vi "SetScrapped.vi"(8 "error in":errorcluster, 10 "Srapped":bool, 11 "ProductUnit in":refnum<class "ProductUnit.lvclass">) -> (0 "error out":errorcluster, 3 "ProductUnit out":refnum<class "ProductUnit.lvclass">)   [LabVIEW 2021, in "ProligentXMLGenerator.lvlib" / "ProductUnit.lvclass"]
doc: "Flag representing whether the product unit has been scrapped or not. When not specified, it is assumed that the product unit is not scrapped."
uses:
  ProductUnit.lvclass
  ProductUnit.lvclass/ProductUnit.ctl
  Base/Attribute/Attribute.lvclass
  Base/Boolean/Boolean.lvclass
  C:/Projects/proligent-xml-generator-labview/src/ProligentXMLGenerator/Base/Attribute/Attribute.lvclass
  Base/DateTime/DateTime.lvclass
  C:/Projects/proligent-xml-generator-labview/src/ProligentXMLGenerator/Base/DateTime/DateTime.lvclass
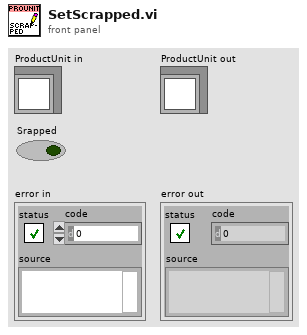
[diagram p1: front panel]
types:
  T1 = typedef "ProligentXMLGenerator.lvlib/ProductUnit.lvclass/Data.ctl" = cluster{"Name":string, "Characteristics":refnum<class "Characteristic.lvclass">[], "Documents":refnum<class "Document.lvclass">[], "CustomData":refnum<class "CustomData.lvclass">, "ProductUnitIdentifier":refnum<class "NonEmptyString_50.lvclass">, "ProductFullName":refnum<class "FullName.lvclass">, "Scrapped":refnum<class "Boolean.lvclass">, "ScrappedTime":refnum<class "DateTime.lvclass">, "CreationTime":refnum<class "DateTime.lvclass">, "ManufacturingTime":refnum<class "DateTime.lvclass">, "ByManufacturer":refnum<class "NonEmptyString_255.lvclass">, "TimeZoneInfoId":string}
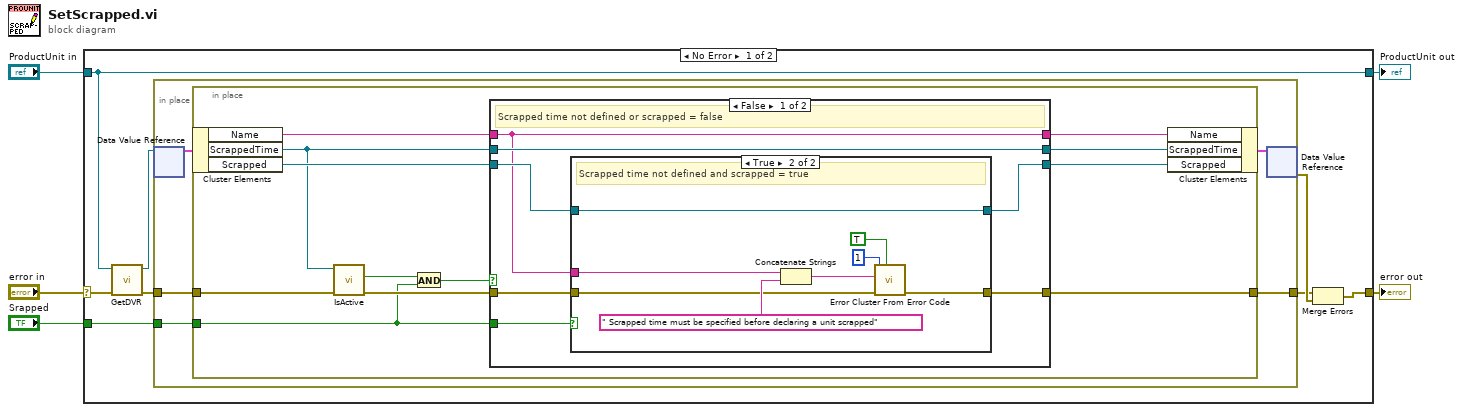
[diagram p0: block diagram]
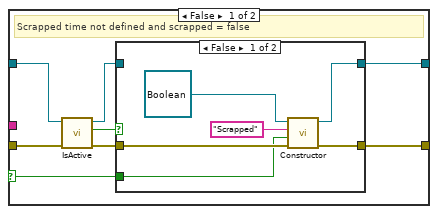
[diagram p2: hidden frame]
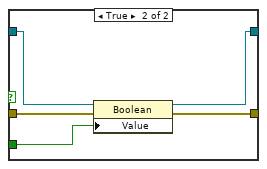
[diagram p3: hidden frame]
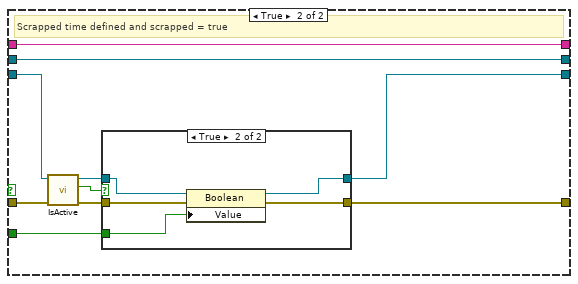
[diagram p4: hidden frame]
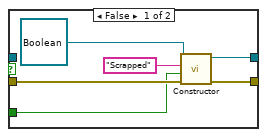
[diagram p5: hidden frame]
diagram:
  n1 = case shown="No Error" "error in" {
    selector: "error in" -> [w11 w86]
    tunnel: "ProductUnit in" -> [w6 w87]
    tunnel: [w8 w86] -> w3
    tunnel: "Srapped" -> [w7 _]
    tunnel: [w6 w87] -> w1
    frame No Error {
      n2 = call "GetDVR.vi"("error in"=w11, "ProductUnit in"=w6) -> ("error out"=w10:errorcluster, "DVRReference"=w12:refnum<data-value>)  [unwired: 8 in]
      n3 = in-place "In Place Element Structure" {
        in-place-border: w10 -> [w18]
        in-place-border: [w17] -> w9
        in-place-border: w7 -> [w16]
        n4 = in-place-dvr #1(w12) -> (w15:T1)  [unwired: 1 out]
        n5 = in-place "In Place Element Structure" {
          in-place-border: w18 -> [w25]
          in-place-border: [w30] -> w17
          in-place-border: w16 -> [w22]
          n6 = in-place-cluster #2(w15) -> ("Name"=w23:string, "ScrappedTime"=w24:refnum<class "DateTime.lvclass">, "Scrapped"=w28:refnum<class "Boolean.lvclass">)
          n7 = call "IsActive.vi"("error in"=w25, "Attribute in"=w24) -> ("error out"=w26:errorcluster, "IsActive"=w21:bool)  [unwired: 7 in, 1 out]
          n8 = And(x=w21, y=w22) -> (x .and. y?=w20:bool)
          n9 = case shown="False" w20 {
            tunnel: [w35 w74] -> w30
            tunnel: w22 -> [w34 w73]
            tunnel: [w33 w72] -> w29
            tunnel: w26 -> [w36 w70]
            tunnel: w28 -> [w32 w69]
            tunnel: [w37 w66] -> w27
            tunnel: w24 -> [w37 w66]
            tunnel: w23 -> [w31 w65]
            tunnel: [w31 w65] -> w19
            frame False {
              # "Scrapped time not defined or scrapped = false"
              n10 = case shown="True" w34 {
                selector: w34 -> [w40 _]
                tunnel: w36 -> [w42 w60]
                tunnel: [w41 w59] -> w35
                tunnel: w31 -> [_ w58]
                tunnel: w32 -> [w39 w57]
                tunnel: [w38 w57] -> w33
                frame False {
                  # "Scrapped time not defined and scrapped = false"
                  n11 = call "IsActive.vi"("error in"=w42, "Attribute in"=w39) -> ("error out"=w45:errorcluster, "IsActive"=w43:bool, "Attribute in"=w44:refnum<class "Boolean.lvclass">)  [unwired: 7 in]
                  n12 = case shown="False" w43 {
                    tunnel: w45 -> [w48 w56]
                    tunnel: [w51 w55] -> w41
                    tunnel: w40 -> [w47 w54]
                    tunnel: [w50 w53] -> w38
                    tunnel: w44 -> [_ w52]
                    frame False {
                      n13 = call-dynamic "Constructor.vi"("error in"=w48, "Value"=w47, "Name"="Scrapped", "Boolean in"=refnum<class "Boolean.lvclass"> refnum ("ProcessVersion")) -> ("error out"=w51:errorcluster, "Boolean out"=w50:refnum<class "Boolean.lvclass">)  [unwired: 6 in]
                    }
                    frame True {
                      n14 = property on="Property Node" class="Boolean"(reference=w52, error in=w56, "Value"=w54) -> (reference out=w53:refnum<class "Boolean.lvclass">, error out=w55:errorcluster)
                    }
                  }
                }
                frame True {
                  # "Scrapped time not defined and scrapped = true"
                  n15 = Concatenate Strings(w58, " Scrapped time must be specified before declaring a unit scrapped" ("string")) -> (w63:string)
                  n16 = call <vilib>:"Error Cluster From Error Code.vi"("show call chain? (False)"=TRUE, "error in (no error)"=w60, "error message (\"\")"=w63, "error code (0)"=1) -> ("error out"=w59:errorcluster)  [unwired: 5 in]
                }
              }
            }
            frame True {
              # "Scrapped time defined and scrapped = true"
              n17 = call "IsActive.vi"("error in"=w70, "Attribute in"=w69) -> ("error out"=w71:errorcluster, "IsActive"=w67:bool, "Attribute in"=w68:refnum<class "Boolean.lvclass">)  [unwired: 7 in]
              n18 = case shown="True" w67 {
                tunnel: w71 -> [w77 w85]
                tunnel: [w80 w84] -> w74
                tunnel: w73 -> [w76 w83]
                tunnel: [w79 w82] -> w72
                tunnel: w68 -> [_ w81]
                frame False {
                  n19 = call-dynamic "Constructor.vi"("error in"=w77, "Value"=w76, "Name"="Scrapped", "Boolean in"=refnum<class "Boolean.lvclass"> refnum ("ProcessVersion")) -> ("error out"=w80:errorcluster, "Boolean out"=w79:refnum<class "Boolean.lvclass">)  [unwired: 6 in]
                }
                frame True {
                  n20 = property on="Property Node" class="Boolean"(reference=w81, error in=w85, "Value"=w83) -> (reference out=w82:refnum<class "Boolean.lvclass">, error out=w84:errorcluster)
                }
              }
            }
          }
          n21 = in-place-cluster #2("Name"=w19, "ScrappedTime"=w27, "Scrapped"=w29) -> (w14:T1)
        }
        n22 = in-place-dvr #1(w14) -> (w13:errorcluster)  [unwired: 1 out]
      }
      n23 = Merge Errors(w9, w13) -> (w8:errorcluster)
    }
    frame Error {
    }
  }
  "error out" <- w3
  "ProductUnit out" <- w1
